vi "KM_HFLI_get_one_data_point -V2.vi.vi"(4 "Oscillator (0)":u16, 8 "Error In":errorcluster, 9 "timeconstant (s)":dbl=0.006, 10 "Freq in (Hz)":dbl=40000.0 format="%#_13g", 11 "Handle In":T1 {"Handle" format="0x%08x"; "Conn" format="0x%08x"}) -> (0 "Error Out":errorcluster, 1 "z out (V)":cdb, 2 "Freq out (Hz)":dbl=40000.0 format="%#_13g", 3 "Handle Out":T1 {"Handle" format="0x%08x"; "Conn" format="0x%08x"})   [LabVIEW 2016]
uses:
  <instrlib>/Zurich Instruments LabOne/Public/ziTypeHandle.ctl
  <instrlib>/Zurich Instruments LabOne/Zurich Instruments LabOne.lvlib
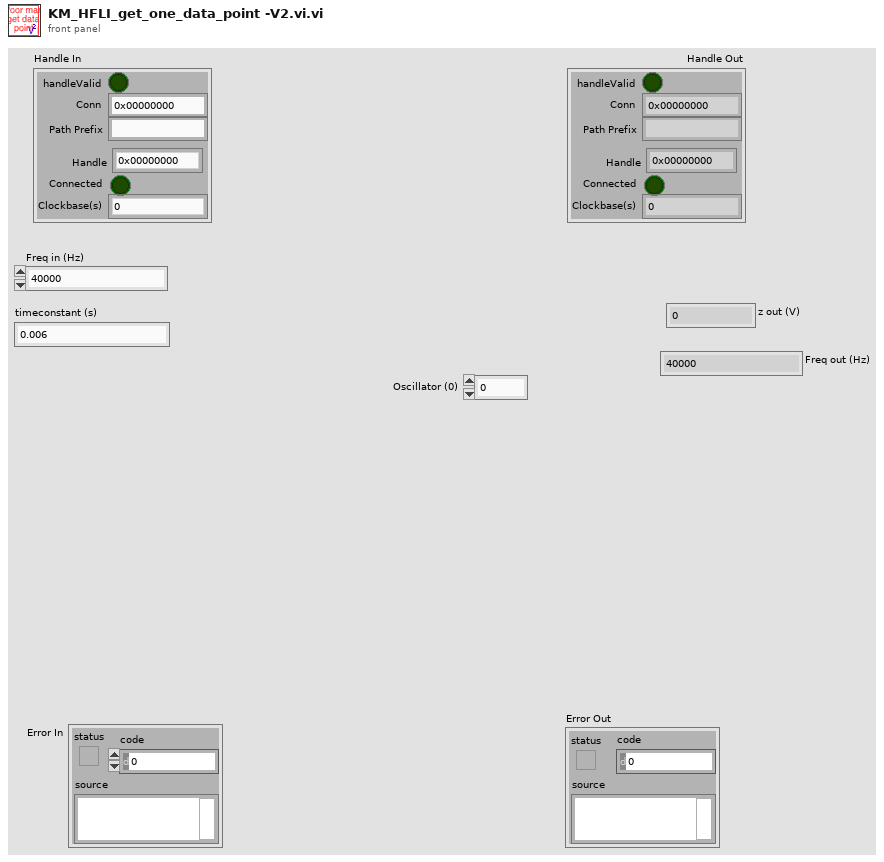
[diagram p1: front panel]
types:
  T1 = typedef "Zurich Instruments LabOne.lvlib/ziTypeHandle.ctl" = cluster{"handleValid":bool, "Conn":u64, "Path Prefix":string, "Handle":u64, "Connected":bool, "Clockbase(s)":dbl}
  T2 = cluster{"Timestamps (ticks)":u64, "X (Vrms)":dbl, "Y (Vrms)":dbl, "Osc Phase (deg)":dbl, "Freq (Hz)":dbl, "DIO":u32, "AuxIn0 (V)":dbl, "AuxIn1 (V)":dbl}
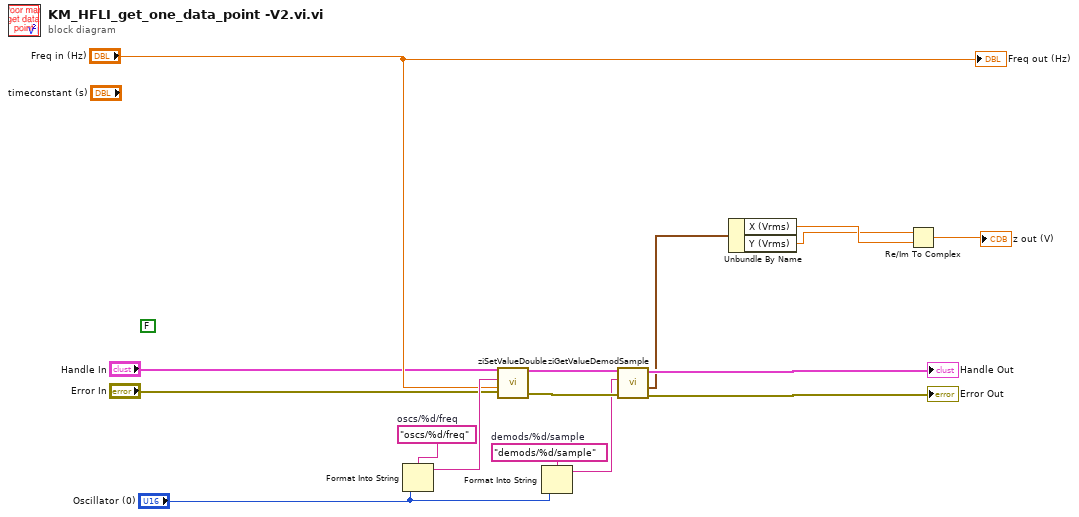
[diagram p0: block diagram]
diagram:
  (unwired) FALSE
  w8 = "demods/%d/sample"  # demods/%d/sample
  w12 = "oscs/%d/freq"  # oscs/%d/freq
  n1 = Format Into String(format string=w12, "Oscillator (0)") -> (resulting string=w11:string)  [unwired: 2 in, 1 out]
  n2 = call <instrlib>:"ziSetValueDouble.vi"("Error In"="Error In", "Value"="Freq in (Hz)", "Path"=w11, "Handle In"="Handle In") -> ("Error Out"=w14:errorcluster, "Handle Out"=w13:T1)  [unwired: 1 in]
  n3 = Format Into String(format string=w8, "Oscillator (0)") -> (resulting string=w9:string)  [unwired: 2 in, 1 out]
  n4 = call <instrlib>:"ziGetValueDemodSample.vi"("error in"=w14, "Path"=w9, "Handle In"=w13) -> ("error out"=→"Error Out":errorcluster, "Demod Sample Out"=w6:T2, "Handle Out"=→"Handle Out":T1)  [unwired: 2 in]
  n5 = Unbundle By Name(w6) -> ("X (Vrms)"=w5:dbl, "Y (Vrms)"=w4:dbl)
  n6 = Re/Im To Complex(1:w5, 2:w4) -> (0:→"z out (V)":cdb)
  "Freq out (Hz)" <- "Freq in (Hz)"
